vi "CleanUp.vi"(8 "error in (no error)":errorcluster, 11 "TestLoader in":refnum<class "TestLoader.lvclass">) -> (0 "error out":errorcluster, 3 "TestLoader out":refnum<class "TestLoader.lvclass">)   [LabVIEW 2013, in "TestLoader.lvclass"]
uses:
  TestLoader.lvclass
panel:
  # "JKI VI Tester for LabVIEW\nhttp://jkisoft.com/vi-tester\nCopyright (C) 2007-2009, JKI <info@jkisoft.com>\nALL RIGHTS RESERVED"
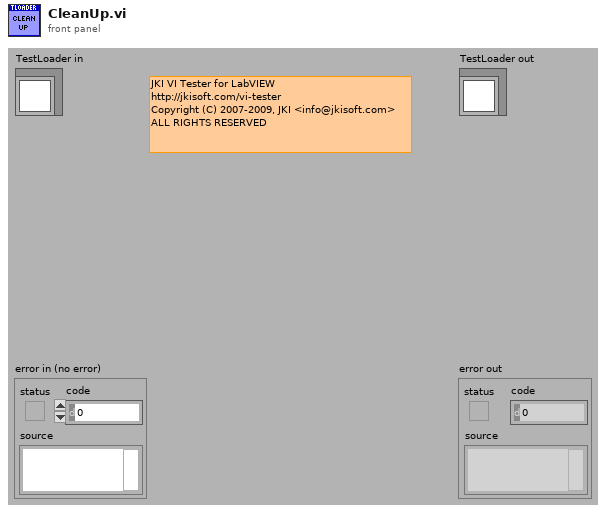
[diagram p1: front panel]
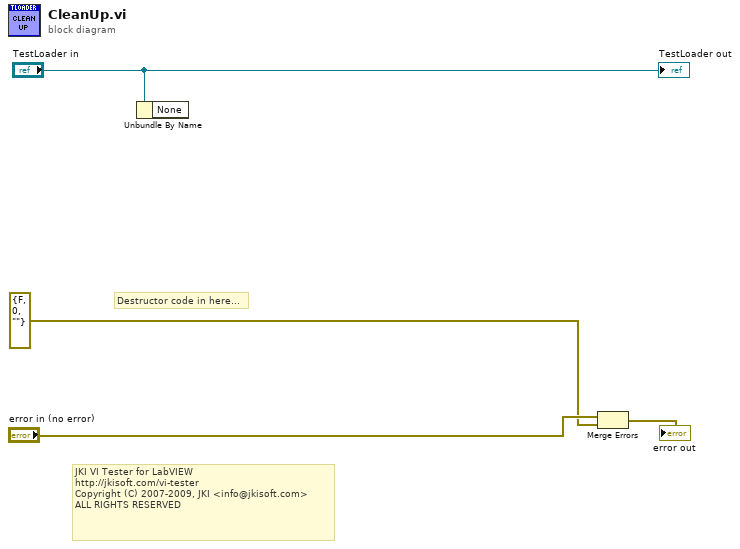
[diagram p0: block diagram]
diagram:
  # "JKI VI Tester for LabVIEW\nhttp://jkisoft.com/vi-tester\nCopyright (C) 2007-2009, JKI <info@jkisoft.com>\nALL RIGHTS RESERVED"
  # "Destructor code in here..."
  n1 = Unbundle By Name("TestLoader in") -> ()  [unwired: 1 out]
  n2 = Merge Errors("error in (no error)", errorcluster {"status"=FALSE, "code"=0, "source"=""} ("error in (no error)")) -> (→"error out":errorcluster)
  "TestLoader out" <- "TestLoader in"
